vi "M to Front Switch.vi"(8 "Command Info In":T1, 10 "M to Front Switch":T4) -> ()   [LabVIEW 2017]
uses:
  Block Clusters/M to Front Switch.ctl
  <vilib>/Rock Robotics/WPI/Framework/Completion Status.ctl
  <vilib>/Rock Robotics/WPI/Framework/Completion Notifier.ctl
  <vilib>/Rock Robotics/WPI/Framework/Command Status Info.ctl
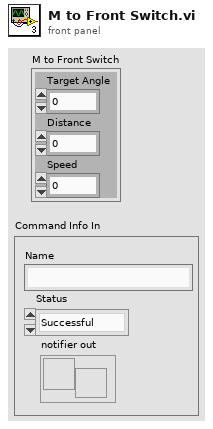
[diagram p1: front panel]
types:
  T1 = typedef "Command Status Info.ctl" = cluster{"Name":string, "Status":T2, "notifier out":T3}
  T2 = typedef "Completion Status.ctl" = enum16{"Successful", "Aborted", "Incomplete"}
  T3 = typedef "Completion Notifier.ctl" = refnum<notifier>
  T4 = typedef "M to Front Switch.ctl" = cluster{"Target Angle":dbl, "Distance":dbl, "Speed":dbl}
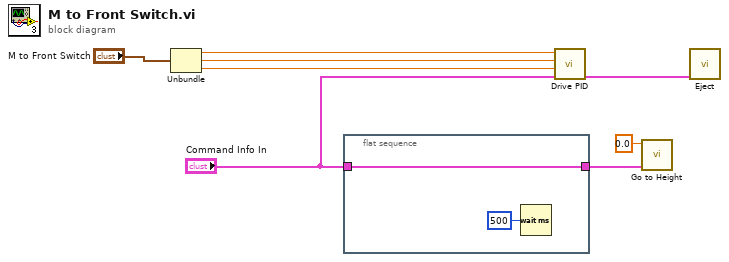
[diagram p0: block diagram]
diagram:
  n1 = Unbundle("M to Front Switch") -> ("Target Angle"=w7:dbl, "Distance"=w6:dbl, "Speed"=w5:dbl)
  n2 = flat-sequence {
    tunnel: "Command Info In" -> [w9]
    tunnel: [w9] -> w3
    frame #0 {
      n3 = Wait (ms)(milliseconds to wait=u32 500) -> ()  [unwired: 1 out]
    }
  }
  n4 = call "Drive PID.vi"("Command Info In"="Command Info In", "Speed"=w5, "Distance"=w6, "Target Angle"=w7) -> ("Command Info Out"=w1:T1)  [unwired: 7 in]
  n5 = call "Go to Height.vi"("Command Info In"=w3, "Target Height (in)"=0.0) -> ()  [unwired: 9 in, 1 out]
  n6 = call "Eject.vi"("Command Info In"=w1) -> ()  [unwired: 10 in, 1 out]
